vi "Pulse_Reset.vi"(2 "error in":errorcluster, 3 "reset?":bool=TRUE, 4 "VISA arduino in":refnum<visa-resource-name>) -> (0 "error out":errorcluster, 1 "VISA arduino out":refnum<visa-resource-name>)   [LabVIEW 2021]
uses:
  Delay_Global.vi
  <vilib>/Utility/error.llb/Error Cluster From Error Code.vi
  <vilib>/ErrorRing/Error Ring.xnode
panel:
  out "delay":u32
  # "Private"
  # "Public"
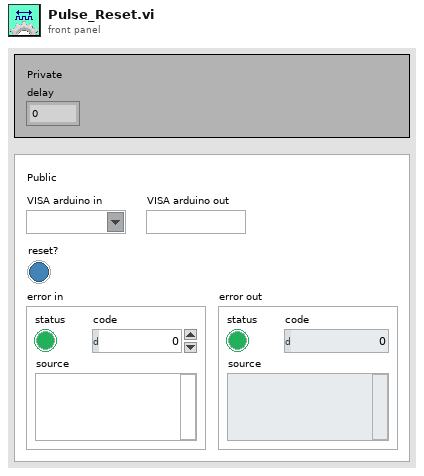
[diagram p1: front panel]
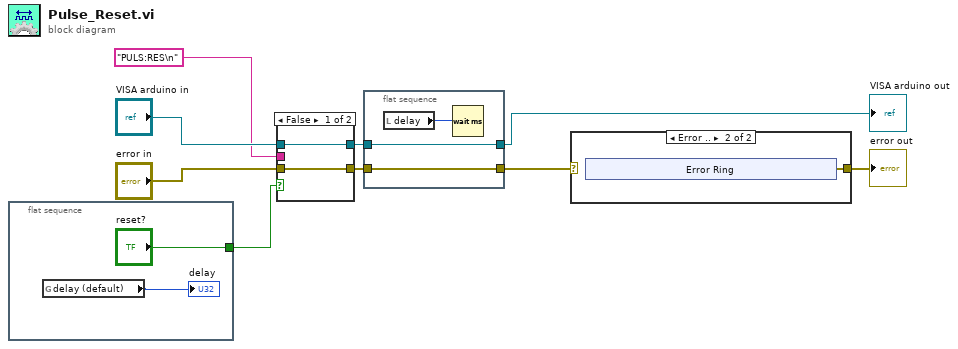
[diagram p0: block diagram]
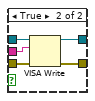
[diagram p2: hidden frame]
diagram:
  n1 = flat-sequence {
    tunnel: ["reset?"] -> w1
    frame #0 {
      n2 = global read "Delay_Global.vi" "delay (default)"() -> (→"delay":u32)
    }
  }
  n3 = case shown="False" w1 {
    tunnel: [w13 w18] -> w8
    tunnel: [w12 w17] -> w7
    tunnel: "VISA arduino in" -> [w13 w16]
    tunnel: "error in" -> [w12 w15]
    tunnel: "PULS:RES\n" -> [_ w14]
    frame False {
    }
    frame True {
      n4 = VISA Write(VISA resource name=w16, write buffer=w14, error in (no error)=w15) -> (VISA resource name out=w18:refnum<visa-resource-name>, error out=w17:errorcluster)  [unwired: 1 out]
    }
  }
  n5 = flat-sequence {
    tunnel: [w21] -> w5
    tunnel: w8 -> [w21]
    tunnel: [w20] -> w9
    tunnel: w7 -> [w20]
    frame #0 {
      n6 = local read "delay"() -> (w19:u32)
      n7 = Wait (ms)(milliseconds to wait=w19) -> ()  [unwired: 1 out]
    }
  }
  n8 = case shown="Error .." w9 {
    selector: w9 -> [w22 _]
    tunnel: [w22 w23] -> w6
    frame No Error {
    }
    frame Error {
      n9 = xnode "Error Ring"() -> ("error out"=w23:errorcluster)
    }
  }
  "error out" <- w6
  "VISA arduino out" <- w5
